vi "toDevVarDoubleStringArray.vi"(1 "ArgIO":cluster{"num data":u8[], "str data":string[]}) -> (0 "argout":cluster{"dvalue":dbl[], "svalue":string[]})   [LabVIEW 2014, in "tango.lvlib"]
uses:
  tango.lvlib
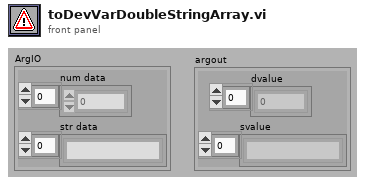
[diagram p1: front panel]
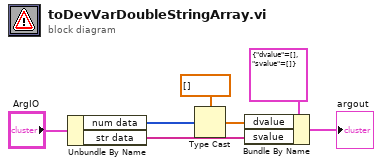
[diagram p0: block diagram]
diagram:
  n1 = Unbundle By Name("ArgIO") -> ("num data"=w5:u8[], "str data"=w2:string[])
  n2 = Type Cast(type=dbl[] [], x=w5) -> (*(type *) &x=w4:dbl[])
  n3 = Bundle By Name(cluster=cluster{"dvalue":dbl[], "svalue":string[]} {"dvalue"=[], "svalue"=[]} ("argin"), "dvalue"=w4, "svalue"=w2) -> (→"argout":cluster{"dvalue":dbl[], "svalue":string[]})
